vi "FreqC.Error handler.vi"(8 "error in":errorcluster, 11 "FreqC Message Session in":T1) -> (0 "error out":errorcluster, 3 "FreqC Message Session out":T1)   [LabVIEW 2018]
uses:
  typedefs/FreqC.Message Session.ctl
  typedefs/FreqC.Message.ctl
  typedefs/FreqC.Message Type.ctl
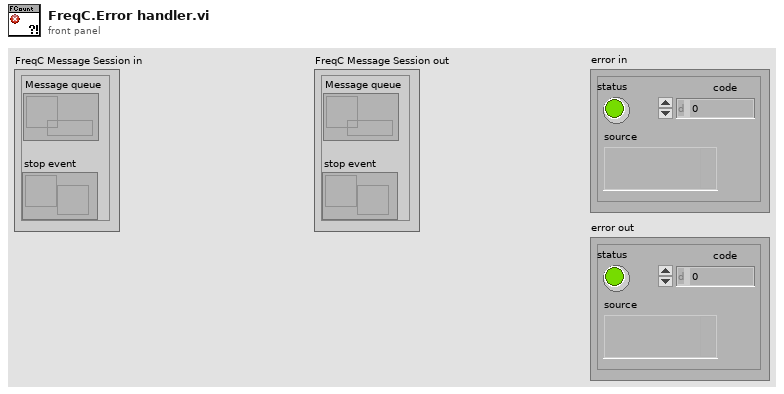
[diagram p1: front panel]
types:
  T1 = typedef "FreqC.Message Session.ctl" = cluster{"Message queue":refnum<queue>, "stop event":refnum<user-event>}
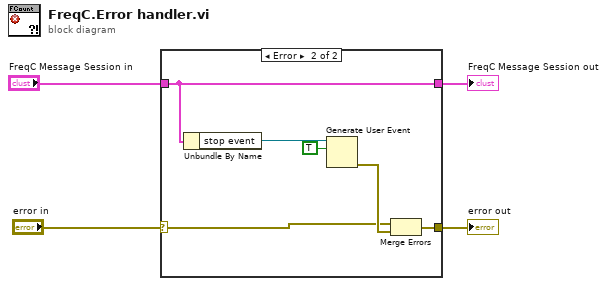
[diagram p0: block diagram]
diagram:
  n1 = case shown="Error" "error in" {
    selector: "error in" -> [w6 w8]
    tunnel: [w6 w7] -> w3
    tunnel: [w5 w12] -> w1
    tunnel: "FreqC Message Session in" -> [w5 w12]
    frame No Error {
    }
    frame Error {
      n2 = Unbundle By Name(w12) -> ("stop event"=w11:refnum<user-event>)
      n3 = Generate User Event(user event=w11, event data cluster=TRUE ("event data")) -> (error out=w9:errorcluster)  [unwired: 2 in, 1 out]
      n4 = Merge Errors(w8, w9) -> (w7:errorcluster)
    }
  }
  "error out" <- w3
  "FreqC Message Session out" <- w1
